vi "Create_MsgQ.vi"(8 "error in (no error)":errorcluster) -> (0 "error out":errorcluster, 3 "Queue out":refnum<queue>)   [LabVIEW 2019, in "MsgQ.lvlib"]
uses:
  MsgQ.lvlib
  TypeDefs/CommandsQ.ctl
  TypeDefs/MsgQ_Commands.ctl
  Service/Service.lvlib
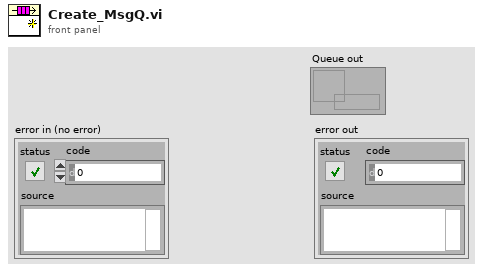
[diagram p1: front panel]
types:
  T1 = typedef "Service.lvlib/CommandsQ.ctl" = cluster{"cmd":T2, "data":variant, "notif":string}
  T2 = typedef "MsgQ.lvlib/MsgQ_Commands.ctl" = enum16{"message1", "message2", "message3", "generic", "transparent", "exception", "stop"}
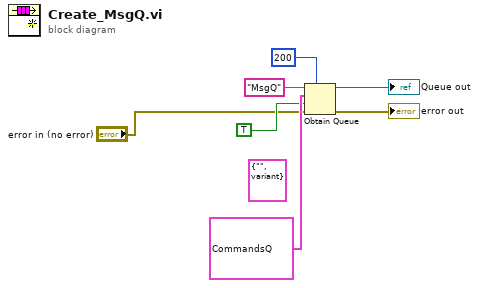
[diagram p0: block diagram]
diagram:
  (unwired) cluster{enum16{""}, "element data type":variant} {enum."", "element data type"=variant}
  n1 = Obtain Queue(max queue size (-1, unlimited)=200, name (unnamed)="MsgQ", element data type=T1 {"cmd"=enum."message1", "data"=variant, "notif"="notif1"}, create if not found? (T)=TRUE, error in (no error)="error in (no error)") -> (queue out=→"Queue out":refnum<queue>, error out=→"error out":errorcluster)  [unwired: 1 out]
